vi "Assert Tree.vi"() -> ()   [LabVIEW 2015, in "BrowerTree.lvclass"]
uses:
  BrowerTree.lvclass
  Type Definition/Symbol Index.ctl
panel:
  out "Navigate Tree:Get Paths":string[](array[string])
  out "BrowerComponentID(\"\")":string
  in  "Tree":string(tree)
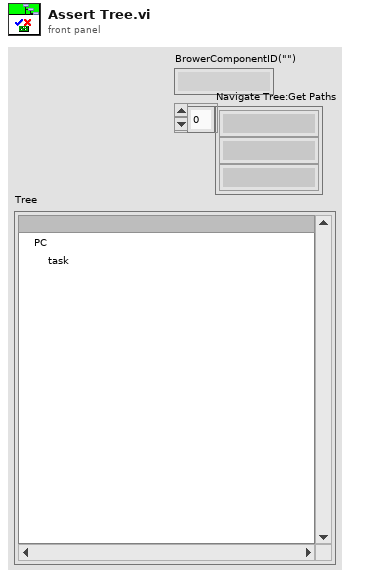
[diagram p1: front panel]
types:
  T1 = typedef "BrowerTree.lvclass/Symbol Index.ctl" = enum16{"PC", "Project", "Module", "DebugTask", "Communication"}
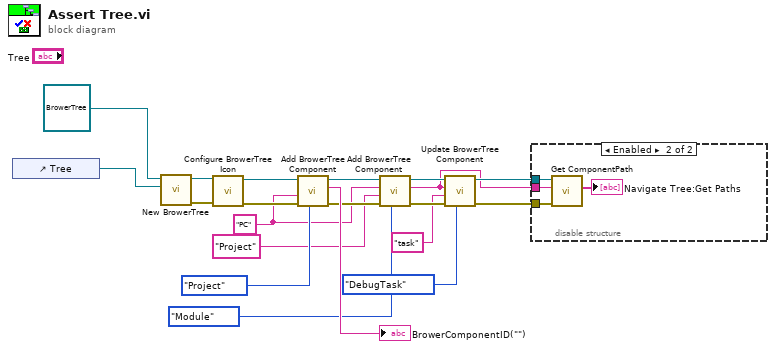
[diagram p0: block diagram]
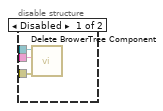
[diagram p2: hidden frame]
diagram:
  w10 = "PC" ("Left Cell String")
  n1 = control-ref of="Tree"() -> (w20:refnum<vi>)
  n2 = call "New BrowerTree.vi"("Tree Refnum"=w20, "BrowerTree in"=refnum<class "BrowerTree.lvclass"> refnum) -> ("error out"=w17:errorcluster, "BrowerTree out"=w18:refnum<class "BrowerTree.lvclass">)  [unwired: 8 in]
  n3 = call "Configure BrowerTree Icon.vi"("error in (no error)"=w17, "BrowerTree in"=w18) -> ("error out"=w15:errorcluster, "BrowerTree out"=w16:refnum<class "BrowerTree.lvclass">)  [unwired: 8 in]
  n4 = call "Add BrowerTree Component.vi"("SymbolIndex"=Symbol_Index."Project", "error in (no error)"=w15, "Left Cell String"=w10, "BrowerTree in"=w16) -> ("error out"=w11:errorcluster, "BrowerComponentID(\"\")"=→"BrowerComponentID(\"\")":string, "BrowerTree out"=w12:refnum<class "BrowerTree.lvclass">)  [unwired: 5 in]
  n5 = call "Add BrowerTree Component.vi"("SymbolIndex"=Symbol_Index."Module", "error in (no error)"=w11, "Left Cell String"="Project", "Parent Tag"=w10, "BrowerTree in"=w12) -> ("error out"=w7:errorcluster, "BrowerComponentID(\"\")"=w1:string, "BrowerTree out"=w8:refnum<class "BrowerTree.lvclass">)  [unwired: 4 in]
  n6 = call "Update BrowerTree Component.vi"("SymbolIndex"=Symbol_Index."DebugTask", "error in (no error)"=w7, "BrowerComponentNewName(\"\")"="task" ("BrowerComponentName(\"\")"), "BrowerComponentID(\"\")"=w1, "BrowerTree in"=w8) -> ("error out"=w5:errorcluster, "BrowerTree out"=w6:refnum<class "BrowerTree.lvclass">)  [unwired: 5 in]
  n7 = disable-structure shown="Enabled" {
    disable-tunnel: w6 -> [w23 w27]
    disable-tunnel: w5 -> [w22 w25]
    disable-tunnel: w1 -> [w21 w26]
    frame Disabled {
      n8 = call "Delete BrowerTree Component.vi"("error in (no error)"=w22, "BrowerComponentID(\"\")"=w21, "BrowerTree in"=w23) -> ()  [unwired: 7 in, 2 out]
    }
    frame Enabled {
      n9 = call "Get ComponentPath.vi"("error in (no error)"=w25, "BrowerComponentID(\"\")"=w26, "BrowerTree in"=w27) -> ("Navigate Tree:Get Paths"=→"Navigate Tree:Get Paths":string[])  [unwired: 6 in, 2 out]
    }
  }
